vi "save_notes.vi"(8 "error in":errorcluster, 9 "Comments":string, 10 "Notes":string[][](table), 11 "ExperimentVariables (in)":refnum<class "ExperimentVariables.lvclass">) -> (0 "error out":errorcluster, 3 "ExperimentVariables":refnum<class "ExperimentVariables.lvclass">)   [LabVIEW 2013]
uses:
  <vilib>/Utility/file.llb/Write To Spreadsheet File (string).vi
  ExperimentVariables/ExperimentVariables.lvclass
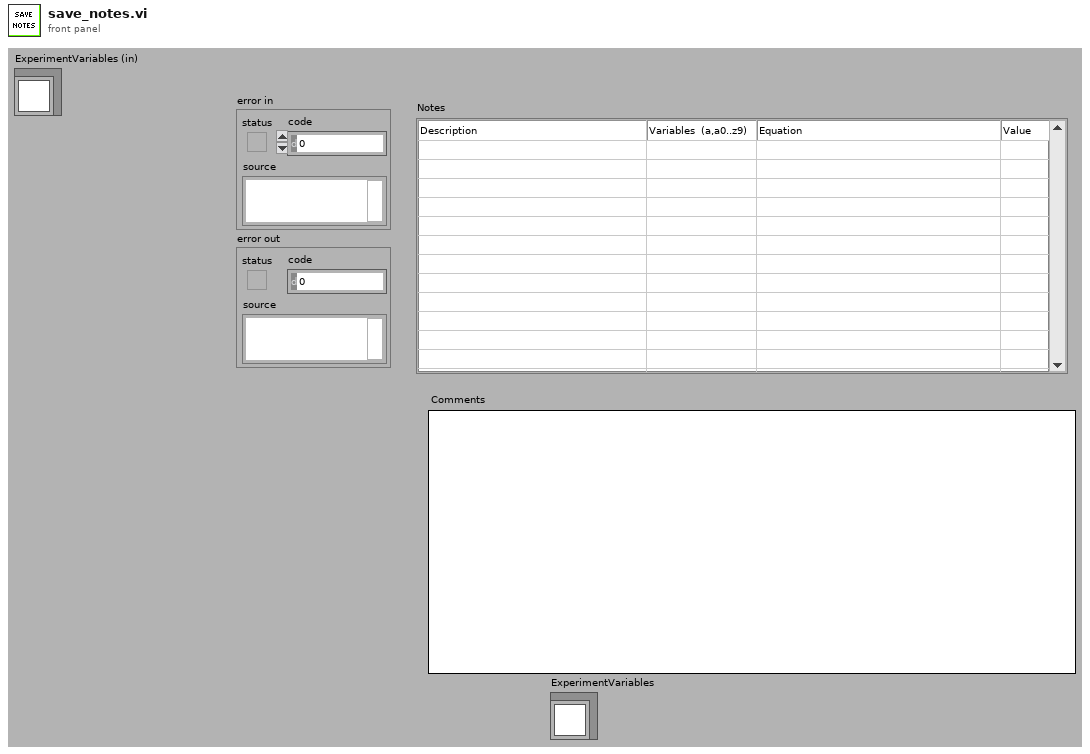
[diagram p1: front panel]
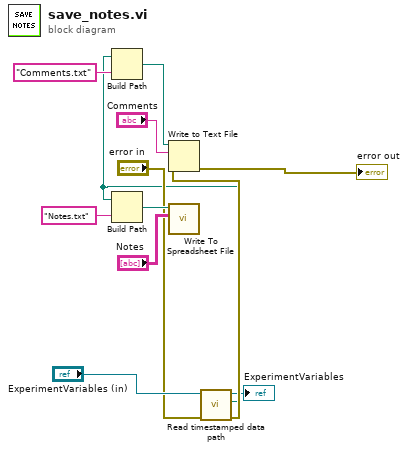
[diagram p0: block diagram]
diagram:
  n1 = call-dynamic "Read timestamped data path.vi"("error in (no error)"="error in", "ExperimentVariables in"="ExperimentVariables (in)") -> ("error out"=w3:errorcluster, "Specific Data Files Path"=w1:path, "ExperimentVariables out"=→"ExperimentVariables":refnum<class "ExperimentVariables.lvclass">)  [unwired: 7 in]
  n2 = Build Path(base path=w1, name or relative path="Comments.txt") -> (appended path=w9:path)
  n3 = Build Path(base path=w1, name or relative path="Notes.txt") -> (appended path=w11:path)
  n4 = Write to Text File(file (use dialog)=w9, text="Comments", error in=w3) -> (error out=→"error out":errorcluster)  [unwired: 1 in, 2 out]
  n5 = call-poly <vilib>:"Write To Spreadsheet File.vi"("2D data"="Notes", "file path (dialog if empty)"=w11) -> ()  [unwired: 6 in, 1 out]
